vi "Time series viewer-Shortcut menu handler.vi"(10 "ItemTag":string) -> ()   [LabVIEW 2017]
uses:
  Typedefs/Speed graph behaviour enum.ctl
  Globals/gl_Time series viewer globals.vi
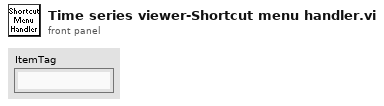
[diagram p1: front panel]
types:
  T1 = typedef "Time series viewer refs.ctl" = cluster{"This VI":refnum<vi>, "Image control":refnum<vi>, "AVI Mode ind":refnum<vi>, "Play":refnum<vi>, "Stop":refnum<vi>, "Back":refnum<vi>, "Scrollbar":refnum<vi>, "Video length info":refnum<vi>, "Expected speed values":refnum<vi>, "Intensity":refnum<vi>, "Path":refnum<vi>, "Selection sliders":refnum<vi>, "Speed Graph ref":refnum<vi>, "Frame rate set (fps)":refnum<vi>, "Channel to load":refnum<vi>, "Number of rows to generate":refnum<vi>, "Colour":refnum<vi>}
  T2 = typedef "Speed graph behaviour enum.ctl" = enum16{"Scrolling data", "Scrolling cursor"}
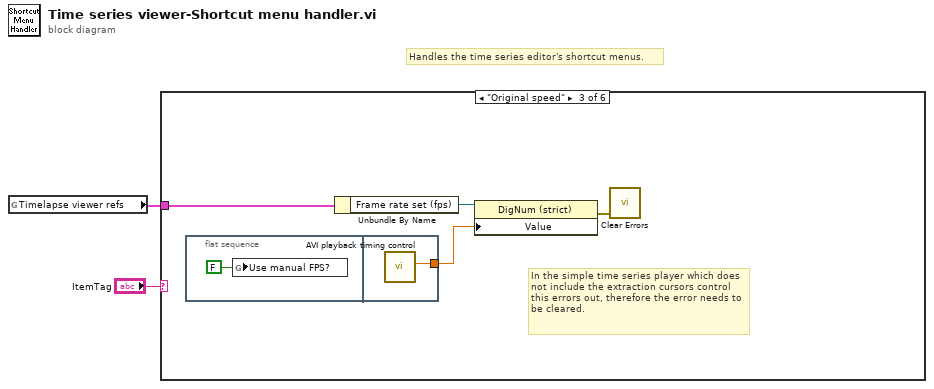
[diagram p0: block diagram]
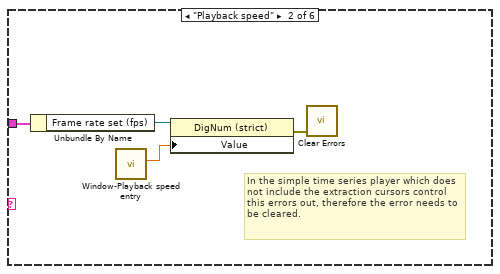
[diagram p3: hidden frame]
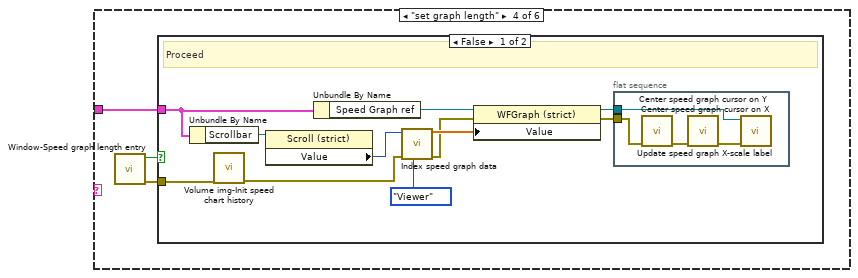
[diagram p4: hidden frame]
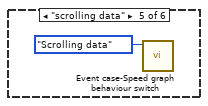
[diagram p6: hidden frame]
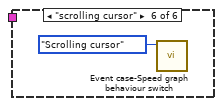
[diagram p7: hidden frame]
diagram:
  # "Handles the time series editor's shortcut menus."
  n1 = global read "gl_Time series viewer globals.vi" "Timelapse viewer refs"() -> (w1:T1)
  n2 = case shown="\"Original speed\"" "ItemTag" {
    tunnel: w1 -> [_ w4 w8 w13 _ _]
    frame Default {
    }
    frame "Playback speed" {
      # "In the simple time series player which does not include the extraction cursors control this errors out, therefore the error needs to be cleared."
      n3 = Unbundle By Name(w4) -> ("Frame rate set (fps)"=w6:refnum<vi>)
      n4 = call "Window-Playback speed entry.vi"() -> ("Frame rate set (fps)"=w5:dbl)  [unwired: 10 in, 1 out]
      n5 = property class="DigNum (strict)"(reference=w6, "Value"=w5) -> (error out=w3:errorcluster)  [unwired: 1 in, 1 out]
      n6 = call <vilib>:"Clear Errors.vi"("error in (no error)"=w3) -> ()  [unwired: 5 in, 2 out]
    }
    frame "Original speed" {
      # "In the simple time series player which does not include the extraction cursors control this errors out, therefore the error needs to be cleared."
      n7 = flat-sequence {
        tunnel: [w12] -> w9
        frame #0 {
          n8 = global write "gl_Time series viewer globals.vi" "Use manual FPS?"(FALSE ("Use manual FPS?")) -> ()
        }
        frame #1 {
          n9 = call "AVI playback timing control.vi"() -> ("Frame rate set OR original (fps)"=w12:dbl)  [unwired: 8 in, 3 out]
        }
      }
      n10 = Unbundle By Name(w8) -> ("Frame rate set (fps)"=w10:refnum<vi>)
      n11 = property class="DigNum (strict)"(reference=w10, "Value"=w9) -> (error out=w7:errorcluster)  [unwired: 1 in, 1 out]
      n12 = call <vilib>:"Clear Errors.vi"("error in (no error)"=w7) -> ()  [unwired: 5 in, 2 out]
    }
    frame "set graph length" {
      n13 = call "Window-Speed graph length entry.vi"() -> ("error out (no error)"=w14:errorcluster, "Cancelled"=w15:bool)  [unwired: 10 in]
      n14 = case shown="False" w15 {
        tunnel: w14 -> [w25 _]
        tunnel: w13 -> [w17 _]
        frame False {
          # "Proceed"
          n15 = Unbundle By Name(w17) -> ("Scrollbar"=w24:refnum<vi>)
          n16 = call "Volume img-Init speed chart history.vi"("error in (no error)"=w25) -> ("error out"=w20:errorcluster)  [unwired: 10 in]
          n17 = property class="Scroll (strict)"(reference=w24) -> ("Value"=w23:i32)  [unwired: 1 in, 2 out]
          n18 = Unbundle By Name(w17) -> ("Speed Graph ref"=w22:refnum<vi>)
          n19 = call "Index speed graph data.vi"("Caller"=enum16{"Viewer", "Exporter"}."Viewer", "error in (no error)"=w20, "Gobal frame number in Timelapse data/master video (1 based)"=w23) -> ("error out"=w18:errorcluster, "Speed data waveform graph"=w26:dbl[])  [unwired: 6 in, 1 out]
          n20 = property class="WFGraph (strict)"(reference=w22, error in=w18, "Value"=w26) -> (reference out=w21:refnum<vi>, error out=w19:errorcluster)
          n21 = flat-sequence {
            tunnel: w21 -> [w28]
            tunnel: w19 -> [w27]
            frame #0 {
              n22 = call "Center speed graph cursor on X.vi"("error in (no error)"=w27) -> ("error out"=w30:errorcluster)  [unwired: 10 in]
              n23 = call "Center speed graph cursor on Y.vi"("error in (no error)"=w30) -> ("error out"=w29:errorcluster)  [unwired: 10 in]
              n24 = call "Update speed graph X-scale label.vi"("error in (no error)"=w29, "Speed Graph"=w28) -> ()  [unwired: 9 in, 1 out]
            }
          }
        }
        frame True {
          # "Cancelled"
        }
      }
    }
    frame "scrolling data" {
      n25 = call "Event case-Speed graph behaviour switch.vi"("Speed graph behaviour"=Speed_graph_behaviour_enum."Scrolling data") -> ()  [unwired: 10 in, 1 out]
    }
    frame "scrolling cursor" {
      n26 = call "Event case-Speed graph behaviour switch.vi"("Speed graph behaviour"=Speed_graph_behaviour_enum."Scrolling cursor") -> ()  [unwired: 10 in, 1 out]
    }
  }
